vi "GetTimeStampFromTimeCtrl.vi"(11 "ref in":refnum<vi>) -> (2 "result":timestamp, 3 "ref out":refnum<vi>)   [LabVIEW 2018, in "Library-Ctrl.lvlib"]
uses:
  Library-Ctrl.lvlib
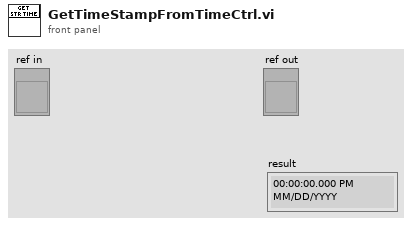
[diagram p1: front panel]
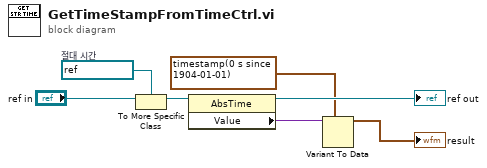
[diagram p0: block diagram]
diagram:
  w6 = refnum<vi> refnum  # 절대 시간
  n1 = To More Specific Class(target class=w6, reference="ref in") -> (specific class reference=w5:refnum<vi>)  [unwired: 1 in, 1 out]
  n2 = property class="AbsTime"(reference=w5) -> (reference out=→"ref out":refnum<vi>, "Value"=w3:variant)  [unwired: 1 in, 1 out]
  n3 = Variant To Data(type=timestamp(0 s since 1904-01-01), Variant=w3) -> (data=→"result":timestamp)  [unwired: 1 in, 1 out]
